vi "Assert Error.vi"(4 "Execution time (s)":dbl=-1.0, 5 "Assert Only? (F)":bool, 6 "error code (1)":i32=1, 7 "Label":string, 8 "error in (no error)":errorcluster, 9 "Register with caller test (F)":bool, 11 "Error?":errorcluster) -> (0 "error out":errorcluster, 2 "Properties.Assert":refnum<class "Properties.Assert.lvclass">)   [LabVIEW 2020, in "Caraya.lvlib" / "Assert.lvclass"]
doc: "Generates an error if the input condition is not met.\n\n--\nCopyright © 2015 JKI All rights reserved.\n\nAuthor: Tomi Maila <tomi.maila@jki.net>\n\nThis library is provided \"AS IS\" ,WITHOUT WARRANTIES OR\nCONDITIONS OF ANY KIND, either express or implied.\n\nJKI -- jki.net"
uses:
  Assert.lvclass
  Properties.Assert/Properties.Assert.lvclass
  C:/projects/caraya/src/classes/Properties/Properties.lvclass
  Properties/Properties.lvclass
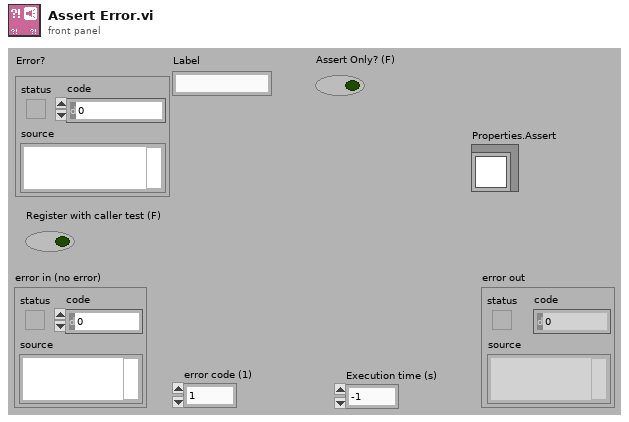
[diagram p1: front panel]
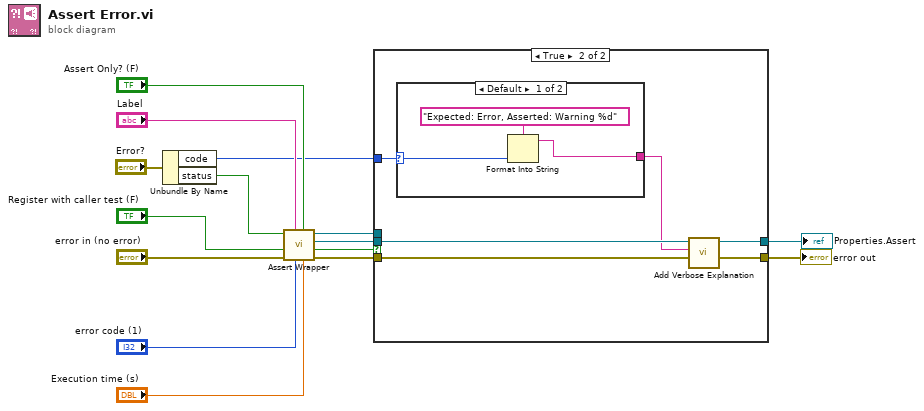
[diagram p0: block diagram]
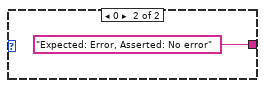
[diagram p3: hidden frame]
diagram:
  n1 = Unbundle By Name("Error?") -> ("code"=w5:i32, "status"=w12:bool)
  n2 = call "Assert Wrapper.vi"("Execution time (s)"="Execution time (s)", "Assert Only? (F)"="Assert Only? (F)", "error code (1)"="error code (1)", "Label"="Label", "error in (no error)"="error in (no error)", "Register with caller test (F)"="Register with caller test (F)", "Assert?"=w12) -> ("error out"=w9:errorcluster, "Verbose"=w6:bool, "Properties.Assert"=w2:refnum<class "Properties.Assert.lvclass">, "Assert out"=w3:refnum<class "Assert.lvclass">)  [unwired: 1 in]
  n3 = case shown="True" w6 {
    tunnel: [w17 w20] -> w7
    tunnel: w3 -> [_ _]
    tunnel: w9 -> [w17 w21]
    tunnel: w5 -> [_ w23]
    tunnel: w2 -> [w16 w22]
    tunnel: [w16 w18] -> w1
    frame False {
    }
    frame True {
      n4 = case shown="Default" w23 {
        selector: w23 -> [w26 _]
        tunnel: [w24 "Expected: Error, Asserted: No error"] -> w19
        frame Default {
          n5 = Format Into String(format string="Expected: Error, Asserted: Warning %d", w26) -> (resulting string=w24:string)  [unwired: 2 in, 1 out]
        }
        frame 0 {
        }
      }
      n6 = call "Add Verbose Explanation.vi"("error in (no error)"=w21, "Verbose Explanation"=w19, "Properties"=w22) -> ("error out"=w20:errorcluster, "Properties"=w18:refnum<class "Properties.Assert.lvclass">)  [unwired: 7 in]
    }
  }
  "error out" <- w7
  "Properties.Assert" <- w1
